vi "Set Retardance.vi"(8 "errorIN":errorcluster caption="Error", 9 "milliseconds to wait (0)":u32, 10 "Retardance":dbl[unit], 11 "LCD in":refnum<class "LCD Retarder.lvclass">) -> (0 "errorOUT":errorcluster caption="Error out", 2 "Retardance out":dbl[unit], 3 "LCD out":refnum<class "LCD Retarder.lvclass">)   [LabVIEW 2017, in "LCD Retarder.lvclass"]
uses:
  LCD Retarder.lvclass
  LCD Retarder.lvclass/LCD Retarder.ctl
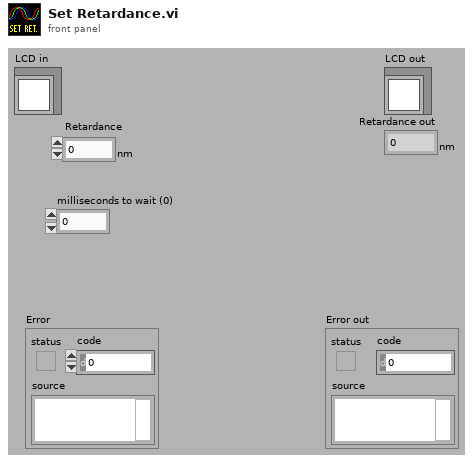
[diagram p1: front panel]
types:
  T1 = cluster{"Device Handle":u32, "Pipe 0 Handle":u32, "Pipe 1 Handle":u32}
  T2 = typedef "Readable.lvclass/X array.ctl" = T3[]
  T3 = typedef "Readable.lvclass/X.ctl" = dbl
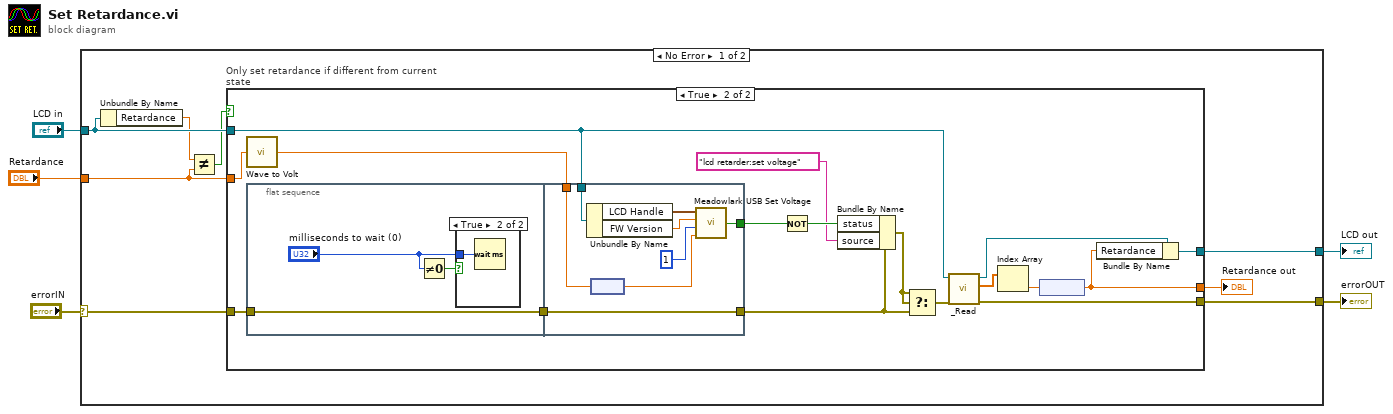
[diagram p0: block diagram]
diagram:
  n1 = case shown="No Error" "errorIN" {
    selector: "errorIN" -> [w12 w46]
    tunnel: "Retardance" -> [w9 _]
    tunnel: "LCD in" -> [w10 w47]
    tunnel: [w11 w47] -> w4
    tunnel: [w13 w46] -> w3
    frame No Error {
      n2 = Unbundle By Name(w10) -> ("Retardance"=w8:dbl[unit])
      n3 = Not Equal?(x=w8, y=w9) -> (x != y?=w7:bool)
      n4 = case "Only set retardance if different from current state" shown="True" w7 {
        tunnel: [w15 w31] -> w13
        tunnel: w12 -> [w15 w25]
        tunnel: [w16 w23] -> w11
        tunnel: w9 -> [w14 w21]
        tunnel: w10 -> [w16 w18]
        tunnel: [w14 w17] -> w6
        frame False {
          # "Only set retardance if different from current state"
        }
        frame True {
          n5 = call "Wave to Volt.vi"("Retardance"=w21) -> ("Voltage"=w20:dbl[unit])
          n6 = flat-sequence {
            tunnel: w25 -> [w36]
            tunnel: [w36] -> w33
            tunnel: [w45] -> w26
            tunnel: w33 -> [w45]
            tunnel: w18 -> [w40]
            tunnel: w20 -> [w39]
            tunnel: [w38] -> w24
            frame #0 {
              n7 = Not Equal To 0?(x="milliseconds to wait (0)") -> (x != 0?=w34:bool)
              n8 = case shown="True" w34 {
                tunnel: "milliseconds to wait (0)" -> [_ w37]
                frame False {
                }
                frame True {
                  n9 = Wait (ms)(milliseconds to wait=w37) -> ()  [unwired: 1 out]
                }
              }
            }
            frame #1 {
              n10 = Unbundle By Name(w40) -> ("LCD Handle"=w43:T1, "FW Version"=w42:dbl)
              n11 = node(w39) -> (w44:dbl)
              n12 = call "Meadowlark USB Set Voltage.VI"("LC Voltage"=w44, "LC Channel"=1, "FW Version"=w42, "USB Open Device Cluster"=w43) -> ("Successful?"=w38:bool)
            }
          }
          n13 = Not(x=w24) -> (.not. x?=w30:bool)
          n14 = Bundle By Name(cluster=w26, "status"=w30, "source"="lcd retarder:set voltage") -> (w29:errorcluster)
          n15 = Select(t=w29, s=w29, f=w26) -> (s? t:f=w28:errorcluster)
          n16 = call-dynamic "_Read.vi"("errorIN"=w28, "LCD in"=w18) -> ("errorOUT"=w31:errorcluster, "X array"=w22:T2, "LCD out"=w32:refnum<class "LCD Retarder.lvclass">)  [unwired: 7 out]
          n17 = Index Array(array=w22) -> (element=w19:T3)  [unwired: 1 in]
          n18 = node(w19) -> (w17:dbl[unit])
          n19 = Bundle By Name(cluster=w32, "Retardance"=w17) -> (w23:refnum<class "LCD Retarder.lvclass">)
        }
      }
      "Retardance out" <- w6
    }
    frame Error {
    }
  }
  "errorOUT" <- w3
  "LCD out" <- w4
